vi "Close Std In.vi"(8 "error in":errorcluster, 11 "ASE Handle":refnum<class "ase.lvclass">) -> (0 "error out":errorcluster, 1 "State":T1, 3 "ASE Handle Duplicate":refnum<class "ase.lvclass">)   [LabVIEW 2020, in "serenial.io-ase.lvlib" / "ase.lvclass"]
doc: "<B>Close the Standard Input.</B>\n\nThis will prevent any further writing to the standard input.\n\n<B>This VI will still operate when there is an error at the error-in terminal.</B>\n\nThis VI generates the following errors:\n-5691000: Internal Library Error. Check Error Message for more details.\n1556: Invalid Handle Supplied"
uses:
  ase.lvclass
  Standard Input State.ctl
  ase.lvclass/ase.ctl
  Error Internal Library Implementation Error.vi
  <vilib>/Utility/error.llb/Error Cluster From Error Code.vi
  serenial.io-ase.32.dll
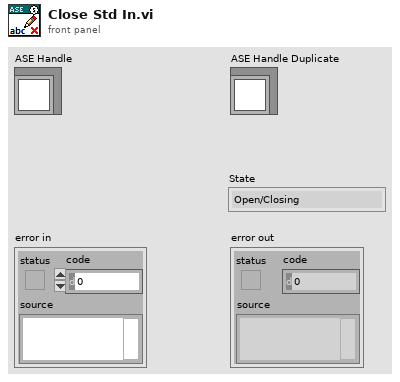
[diagram p1: front panel]
types:
  T1 = typedef "serenial.io-ase.lvlib/ase.lvclass/Standard Input State.ctl" = enum16{"Open/Closing", "Closed"}
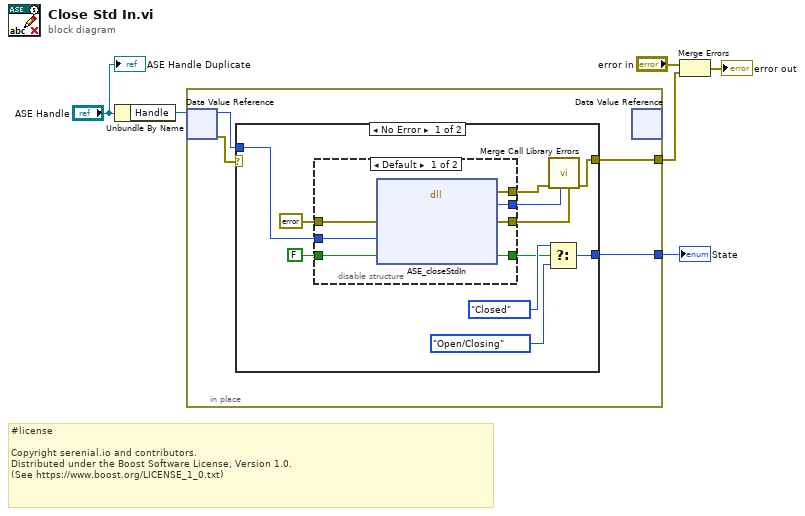
[diagram p0: block diagram]
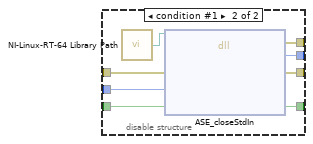
[diagram p2: hidden frame]
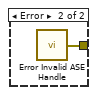
[diagram p3: hidden frame]
diagram:
  # "#license\n\nCopyright serenial.io and contributors.\nDistributed under the Boost Software License, Version 1.0.\n(See https://www.boost.org/LICENSE_1_0.txt)"
  n1 = Unbundle By Name("ASE Handle") -> ("Handle"=w3:refnum<data-value>)
  n2 = in-place "In Place Element Structure" {
    in-place-border: [w9] -> w6
    in-place-border: [w8] -> w4
    n3 = in-place-dvr #1(w3) -> (w7:u64, w10:errorcluster)
    n4 = case shown="No Error" w10 {
      tunnel: w7 -> [w16 _]
      tunnel: [w21 w37] -> w9
      tunnel: [w18 _] -> w8
      frame No Error {
        n5 = disable-structure shown="Default" {
          disable-tunnel: errorcluster {"status"=FALSE, "code"=0, "source"=""} ("error") -> [w28 w36]
          disable-tunnel: w16 -> [w27 w35]
          disable-tunnel: FALSE -> [w26 w34]
          disable-tunnel: [w25 w32] -> w14
          disable-tunnel: [w24 w31] -> w13
          disable-tunnel: [w23 w29] -> w12
          disable-tunnel: [w22 w30] -> w11
          frame condition #0 (active) {
            n6 = dll-call lib="C:/serenial/libraries/Asynchronous-System-Executive/LabVIEW/serenial.io-ase/ase/serenial.io-ase.*.*" fn="ASE_closeStdIn"("Error Out"=w28, "ASE interface"=w27, "Already Closed"=w26) -> (error out=w25:errorcluster, "Error Code"=w24:i32, "Error Out"=w23:errorcluster, "Already Closed"=w22:bool)  [unwired: 4 in, 1 out]
          }
          frame condition #1 {
            n7 = call "NI-Linux-RT-64 Library Path.vi"() -> ("Path"=w33:path)
            n8 = dll-call lib="?" fn="ASE_closeStdIn"(path in=w33, "Error Out"=w36, "ASE interface"=w35, "Already Closed"=w34) -> (error out=w32:errorcluster, "Error Code"=w31:i32, "Error Out"=w29:errorcluster, "Already Closed"=w30:bool)  [unwired: 3 in, 1 out]
          }
        }
        n9 = Select(t=Standard_Input_State."Closed", s=w11, f=Standard_Input_State."Open/Closing" ("State")) -> (s? t:f=w18:T1)
        n10 = call "Merge Call Library Errors.vi"("Library Call Returned Error"=w12, "Error Code"=w13, "error in"=w14) -> ("error IO"=w21:errorcluster)  [unwired: 8 in]
      }
      frame Error {
        n11 = call "Error Invalid ASE Handle.vi"() -> ("Invalid ASE Handle"=w37:errorcluster)
      }
    }
    n12 = in-place-dvr #1() -> ()  [unwired: 1 in, 2 out]
  }
  "State" <- w4
  n13 = Merge Errors("error in", w6) -> (→"error out":errorcluster)
  "ASE Handle Duplicate" <- "ASE Handle"
